vi "Robot Globals.vi"() -> ()   [LabVIEW 2019]
panel:
  in  "Shooter Velocity":dbl
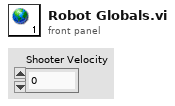
[diagram p1: front panel]
diagram:
